vi "tcp_write.vi"(8 "error in (no error)":errorcluster, 9 "ms_timeout":i32, 10 "data in":string, 11 "conn in":refnum<k5>) -> (0 "error out":errorcluster, 3 "conn out":refnum<k5>)   [LabVIEW 2017, in "rethinkdb.lvlib"]
uses:
  rethinkdb.lvlib
  debug_action.ctl
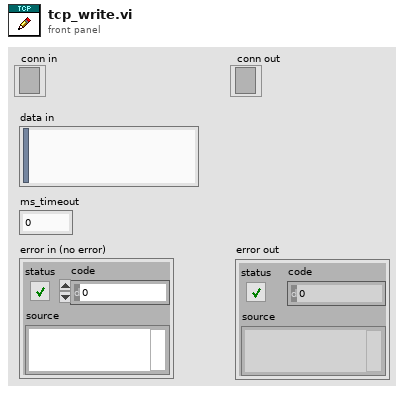
[diagram p1: front panel]
types:
  T1 = typedef "rethinkdb.lvlib/debug_action.ctl" = enum8{"get", "set_query", "set_response", "clear"}
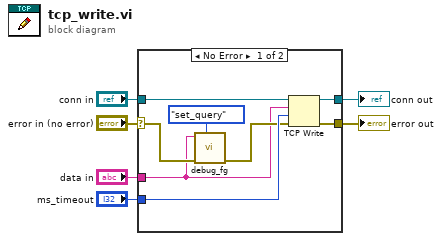
[diagram p0: block diagram]
diagram:
  n1 = case shown="No Error" "error in (no error)" {
    selector: "error in (no error)" -> [w10 w16]
    tunnel: "ms_timeout" -> [w14 _]
    tunnel: [w13 w15] -> w5
    tunnel: "data in" -> [w7 _]
    tunnel: [w12 w16] -> w3
    tunnel: "conn in" -> [w11 w15]
    frame No Error {
      n2 = call "debug_fg.vi"("action"=debug_action."set_query", "error in (no error)"=w10, "data"=w7) -> ("error out"=w9:errorcluster)  [unwired: 7 in, 1 out]
      n3 = TCP Write(connection ID=w11, data in=w7, error in (no error)=w9, 9:w14) -> (connection ID out=w13:refnum<k5>, error out=w12:errorcluster)  [unwired: 1 out]
    }
    frame Error {
    }
  }
  "conn out" <- w5
  "error out" <- w3
